vi "GetCurrentInfo.vi"(0 "reference in":refnum<class "MediaPlayer.lvclass">, 11 "Error In":errorcluster) -> (4 "reference out":refnum<class "MediaPlayer.lvclass">, 8 "Current Info":T1, 15 "Error Out":errorcluster)   [LabVIEW 2024, in "MediaPlayer.lvclass"]
uses:
  MediaPlayer.lvclass
  typedefs/Current Info.ctl
  MediaPlayer.lvclass/MediaPlayer.ctl
panel:
  # "Connector Pane"
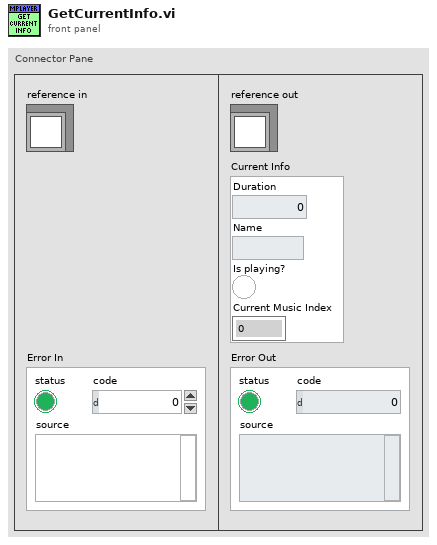
[diagram p1: front panel]
types:
  T1 = typedef "MediaPlayer.lvclass/Current Info.ctl" = cluster{"Duration":dbl, "Name":string, "Is playing?":bool, "Current Music Index":i64}
  T2 = typedef "MediaPlayer.lvclass/ObjectAttributes.ctl" = cluster{"MediaPlayerData":T3, "Current Info":T1}
  T3 = typedef "MediaPlayer.lvclass/MediaPlayer Data.ctl" = cluster{"Music List":path[], "Current Music Index":i64, "Song Handler":T4, "Device ID":u32}
  T4 = typedef "Sound Output Task ID.ctl" = u32
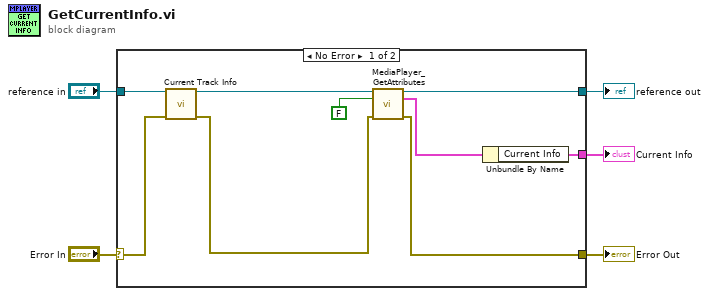
[diagram p0: block diagram]
diagram:
  n1 = case shown="No Error" "Error In" {
    selector: "Error In" -> [w14 w16]
    tunnel: [w13 w16] -> w4
    tunnel: [w12 w15] -> w2
    tunnel: "reference in" -> [w9 w15]
    tunnel: [w6 _] -> w1
    frame No Error {
      n2 = call-dynamic "Current Track Info.vi"("reference in"=w9, "Error In"=w14) -> ("reference out"=w8:refnum<class "MediaPlayer.lvclass">, "Error Out"=w10:errorcluster)  [unwired: 12 in]
      n3 = call "MediaPlayer_GetAttributes.vi"("reference in"=w8, "OnlyGetDvrReference(False)"=FALSE, "Error In"=w10) -> ("reference out"=w12:refnum<class "MediaPlayer.lvclass">, "Data"=w7:T2, "Error Out"=w13:errorcluster)  [unwired: 9 in, 1 out]
      n4 = Unbundle By Name(w7) -> ("Current Info"=w6:T1)
    }
    frame Error {
    }
  }
  "Error Out" <- w4
  "reference out" <- w2
  "Current Info" <- w1
